vi "To Variant.vi"(0 "Obj in":refnum<class "File.lvclass">, 11 "error in (no error)":errorcluster) -> (4 "Obj out":refnum<class "File.lvclass">, 8 "Array":variant[](array[variant]), 15 "error out":errorcluster)   [LabVIEW 2020, in "File.lvclass"]
uses:
  File.lvclass
  File.lvclass/File.ctl
  Waveform/Waveform.lvclass
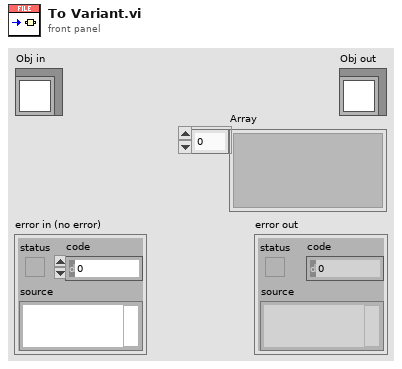
[diagram p1: front panel]
types:
  T1 = typedef "File.lvclass/Serialized.ctl" = cluster{"Filename":path, "Channel":i32, "Loop":bool}
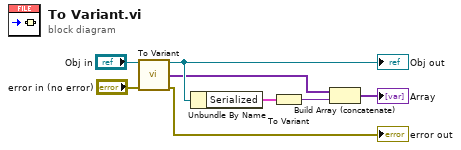
[diagram p0: block diagram]
diagram:
  n1 = call-parent "To Variant.vi"("Obj in"="Obj in", "error in (no error)"="error in (no error)") -> ("Obj out"=w3:refnum<class "File.lvclass">, "Array"=w2:variant[], "error out"=→"error out":errorcluster)  [unwired: 11 in]
  "Obj out" <- w3
  n2 = Unbundle By Name(w3) -> ("Serialized"=w4:T1)
  n3 = To Variant(anything=w4) -> (Variant=w5:variant)
  n4 = Build Array (concatenate)(w2, w5) -> (→"Array":variant[])
